vi "Disable Default File.vi"(8 "Error In":errorcluster) -> (0 "Error Out":errorcluster)   [LabVIEW 2015, in "Logger.lvlib"]
doc: "Turns off, or disables, the internal, default log file."
uses:
  Logger.lvlib
  Private/File/Action.ctl
  Private/File/File.lvlib
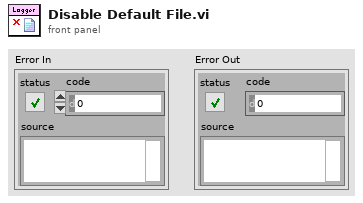
[diagram p1: front panel]
types:
  T1 = typedef "Logger.lvlib/File.lvlib/Action.ctl" = enum16{"Initialize", "Set Maximum File Size", "Set Maximum File Count", "Set Root Folder", "Set Enable Calendar Folder Tree", "Set File Extension", "Start", "Write", "Stop", "Shutdown"}
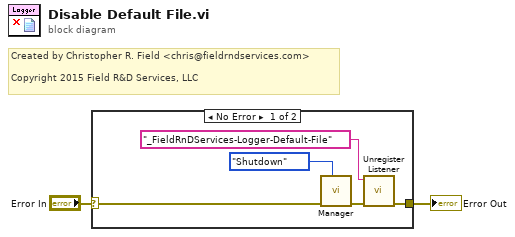
[diagram p0: block diagram]
diagram:
  # "Created by Christopher R. Field <chris@fieldrndservices.com>\n\nCopyright 2015 Field R&D Services, LLC"
  n1 = case shown="No Error" "Error In" {
    selector: "Error In" -> [w7 w8]
    tunnel: [w6 w8] -> w1
    frame No Error {
      n2 = call "Manager.vi"("Action"=Action."Shutdown", "Error In"=w7) -> ("Error Out"=w5:errorcluster)  [unwired: 9 in]
      n3 = call "Unregister Listener.vi"("Error In"=w5, "Listener ID"="_FieldRnDServices-Logger-Default-File") -> ("Error Out"=w6:errorcluster)  [unwired: 9 in]
    }
    frame Error {
    }
  }
  "Error Out" <- w1
